vi "HFRR ADV v06.vi"() -> ()   [LabVIEW 2025] (continued)
                        w3346 = dbl[] [] ("History Data")
                        w3347 = cluster{"y":dbl, dbl, "y":dbl}[] [] ("History Data")
                        w3348 = FALSE ("Visible")
                        n2284 = property on="Stroke ( mm )" class="WFChart (strict)"("History Data"=w3347) -> ()  [unwired: 2 in, 2 out]
                        n2285 = property on="Humidity ( %RH )" class="WFChart (strict)"("History Data"=w3346) -> ()  [unwired: 2 in, 2 out]
                        n2286 = property on="Temperature ( Deg C )" class="WFChart (strict)"("History Data"=w3346) -> ()  [unwired: 2 in, 2 out]
                        n2287 = property on="Electrical Contact Resistance ( % )" class="WFChart (strict)"("History Data"=w3346) -> ()  [unwired: 2 in, 2 out]
                        n2288 = property on="Coefficient of Friction" class="WFChart (strict)"("History Data"=w3346) -> ()  [unwired: 2 in, 2 out]
                        n2289 = property on="Frictional Force ( N )" class="WFChart (strict)"("History Data"=w3346) -> ()  [unwired: 2 in, 2 out]
                        n2290 = property on="Coefficient of Friction" class="WFChart (strict)"("History Data"=w3346) -> ()  [unwired: 2 in, 2 out]
                        n2291 = property on="Frictional Force ( N )" class="WFChart (strict)"("History Data"=w3346) -> ()  [unwired: 2 in, 2 out]
                        n2292 = property on="Electrical Contact Resistance ( % )" class="WFChart (strict)"("History Data"=w3346) -> ()  [unwired: 2 in, 2 out]
                        n2293 = property on="Humidity ( %RH )" class="WFChart (strict)"("History Data"=w3346) -> ()  [unwired: 2 in, 2 out]
                        n2294 = property on="Stroke ( mm )" class="WFChart (strict)"("History Data"=w3347) -> ()  [unwired: 2 in, 2 out]
                        n2295 = property on="Temperature ( Deg C )" class="WFChart (strict)"("History Data"=w3346) -> ()  [unwired: 2 in, 2 out]
                        n2296 = property on="Service Password Log" class="Str"("Visible"=w3348) -> ()  [unwired: 2 in, 2 out]
                        n2297 = property on="Password 3" class="Clust (strict)"("Visible"=w3348) -> ()  [unwired: 2 in, 2 out]
                      }
                    }
                    "TEST FILE NAM,E SAVED" <- TRUE ("TEST FILE NAM,E SAVED")
                  }
                }
              }
            }
          }
        }
        n2298 = case shown="True" w2660 {
          frame False {
            n2299 = local write "tfalg"(0.0 ("tfalg")) -> ()
          }
          frame True {
            n2300 = local read "tfalg"() -> (w2805:dbl)
            n2301 = Equal?(x=w2805, y=0.0) -> (x = y?=w2806:bool)
            n2302 = case shown="True" w2806 {
              frame False {
              }
              frame True {
                n2303 = local read "Total No. of Tests"() -> (w2809:dbl)
                n2304 = local write "tfalg"(1.0 ("tfalg")) -> ()
                n2305 = local write "acq 2"(FALSE ("acq 2")) -> ()
                n2306 = Wait (ms)(milliseconds to wait=u32 200) -> ()  [unwired: 1 out]
                n2307 = Increment(x=w2809) -> (x+1=w2808:dbl)
                n2308 = local write "Total No. of Tests"(w2808) -> ()
              }
            }
          }
        }
        n2309 = local write "Test \nStatus"(w2666) -> ()
        n2310 = local write "Save"(w2666) -> ()
        n2311 = local read "Main Tab"() -> (w2623:T2)
        n2312 = case shown="True" w2647 {
          tunnel: [FALSE ("RUN") TRUE ("RUN")] -> w2646
          tunnel: [_ 1] -> w2639
          frame False {
          }
          frame True {
          }
        }
        n2313 = In Range and Coerce(upper limit=w2654, x=w2627, lower limit=w2653) -> (In Range?=w2645:bool)  [unwired: 1 out]
        n2314 = In Range and Coerce(upper limit=w2651, x=w2626, lower limit=w2652) -> (In Range?=w2643:bool)  [unwired: 1 out]
        n2315 = case shown="True" w2659 {
          frame False {
            n2316 = local read "Rt 3"() -> (w2787:bool)
            n2317 = case shown="True" w2787 {
              frame False {
              }
              frame True {
                n2318 = local write "Rt 3"(FALSE ("Rt 3")) -> ()
                n2319 = local write "Json End Flg"(TRUE ("Upld AR 2")) -> ()
              }
            }
            "Rt" <- TRUE ("Rt")
            "Rt 2" <- FALSE ("Rt")
          }
          frame True {
            n2320 = local read "Rt"() -> (w2794:bool)
            n2321 = local write "Rt 2"(TRUE ("Rt 2")) -> ()
            n2322 = case shown="True" w2794 {
              frame False {
              }
              frame True {
                w2795 = TRUE ("Upld AR 2")
                n2323 = local write "Rt"(FALSE ("Rt")) -> ()
                n2324 = local write "Upld AR"(w2795) -> ()
                n2325 = local write "Json St Flg"(w2795) -> ()
              }
            }
            "Rt 3" <- TRUE ("Rt 3")
          }
        }
        n2326 = case shown="True" w2645 {
          tunnel: [FALSE ("RUN") TRUE ("RUN")] -> w2644
          tunnel: [_ 2] -> w2638
          frame False {
          }
          frame True {
          }
        }
        n2327 = case shown="True" w2643 {
          tunnel: [FALSE ("RUN") TRUE ("RUN")] -> w2642
          tunnel: [_ 3] -> w2637
          frame False {
          }
          frame True {
          }
        }
        n2328 = case shown="\"Acquire\"" w2623 {
          tunnel: w2625 -> [_ w2856]
          frame Default {
            w2855 = 0.0 ("output")
            n2329 = local write "PID-out"(w2855) -> ()
            n2330 = local write "Frequency ( Hz )"(w2855) -> ()
          }
          frame "Acquire" {
            n2331 = stacked-sequence {
              frame #0 {
                n2332 = local read "Auto Start Test"() -> (w2861:bool)
                n2333 = case shown="True" w2861 {
                  tunnel: "RUN" -> [w2881 w2884]
                  tunnel: [w2881 w2883] -> w2862
                  frame False {
                  }
                  frame True {
                    n2334 = local read "Auto Start Temp"() -> (w2882:bool)
                    n2335 = Or(x=w2884, y=w2882) -> (x .or. y?=w2883:bool)
                  }
                }
                n2336 = local read "clk"() -> (w2880:dbl)
                n2337 = local read "Save"() -> (w2876:bool)
                n2338 = Equal?(x=w2880, y=0.0) -> (x = y?=w2877:bool)
                n2339 = And(x=w2877, y=w2876) -> (x .and. y?=w2878:bool)
                n2340 = Not(x="Engage") -> (.not. x?=w2867:bool)
                n2341 = case shown="True" w2862 {
                  tunnel: [0.0 w2901] -> w2859
                  frame False {
                    (unwired) TRUE ("Visible")
                    n2342 = local read "Auto Start Test"() -> (w2888:bool)
                    n2343 = local write "Start Time"(TRUE ("Start Time")) -> ()
                    n2344 = property on="Stroke 2" class="DigNum (strict)"("Visible"=FALSE) -> ()  [unwired: 2 in, 2 out]
                    n2345 = case shown="False" w2888 {
                      frame False {
                        n2346 = property on="Heater Button" class="Bool (strict)"("DisabledEnum"=T15."Enabled" ("Disabled")) -> ()  [unwired: 2 in, 2 out]
                        n2347 = property on="Humidity" class="Bool (strict)"("DisabledEnum"=T15."Enabled" ("Disabled")) -> ()  [unwired: 2 in, 2 out]
                      }
                      frame True {
                      }
                    }
                    n2348 = case shown="False" "TestCompFlg" {
                      frame False {
                        n2349 = local read "StartFlg"() -> (w2896:bool)
                        n2350 = case shown="True" w2896 {
                          frame False {
                          }
                          frame True {
                            n2351 = flat-sequence {
                              frame #0 {
                                n2352 = local read "EVENT LOG"() -> (w2898:string)
                                n2353 = call "Event Log.vi"("Content"="Test was interrupted", "EVENT LOG"=w2898) -> ("EVENT LOG"=w2899:string)  [unwired: 8 in, 1 out]
                                n2354 = local write "EVENT LOG"(w2899) -> ()
                              }
                              frame #1 {
                                w2900 = FALSE ("StartFlg")
                                n2355 = local write "Heater Button"(w2900) -> ()
                                n2356 = local write "StartFlg"(w2900) -> ()
                                n2357 = local write "Humidity"(w2900) -> ()
                              }
                            }
                          }
                        }
                      }
                      frame True {
                      }
                    }
                    n2358 = local write "String 14"("Test will autostart once parameters reach the set value." ("String 14")) -> ()
                  }
                  frame True {
                    (unwired) FALSE ("Visible")
                    n2359 = property on="Stroke 2" class="DigNum (strict)"("Visible"=TRUE) -> ()  [unwired: 2 in, 2 out]
                    n2360 = property on="STOP 2" class="Bool (strict)"("Disabled"=u8 2) -> ()  [unwired: 2 in, 2 out]
                    n2361 = local write "String 14"(" Running....." ("String 14")) -> ()
                    n2362 = property on="Heater Button" class="Bool (strict)"("DisabledEnum"=T15."Disabled and Grayed Out" ("Disabled")) -> ()  [unwired: 2 in, 2 out]
                    n2363 = property on="Humidity" class="Bool (strict)"("DisabledEnum"=T15."Disabled and Grayed Out" ("Disabled")) -> ()  [unwired: 2 in, 2 out]
                    n2364 = case shown="True" "Start Time" {
                      selector: "Start Time" -> [_ w2914]
                      frame False {
                      }
                      frame True {
                        n2365 = Not(x=w2914) -> (.not. x?=w2913:bool)
                        n2366 = local write "Start Time"(w2913) -> ()
                        n2367 = local read "EVENT LOG"() -> (w2915:string)
                        n2368 = call "Event Log.vi"("Content"="Test in progress", "EVENT LOG"=w2915) -> ("EVENT LOG"=w2917:string)  [unwired: 8 in, 1 out]
                        n2369 = local write "EVENT LOG"(w2917) -> ()
                      }
                    }
                    n2370 = local read "Set Hz"() -> (w2911:dbl)
                    n2371 = call <vilib>:"Uniform White Noise Waveform.vi"() -> ("signal out"=w2910:waveform(dbl))  [unwired: 10 in, 1 out]
                    n2372 = Add(x=w2911, y=w2910) -> (x+y=w2909:waveform(dbl))
                    n2373 = Multiply(x=w2909, y=ext 0.1) -> (x*y=w2901:waveform(ext))
                    "StartFlg" <- TRUE ("StartFlg")
                  }
                }
                n2374 = case shown="True" w2878 {
                  frame False {
                  }
                  frame True {
                    n2375 = local write "clk"(10.0 ("clk")) -> ()
                    n2376 = Get Date/Time In Seconds() -> (seconds since 1Jan1904=w2920:timestamp)
                    n2377 = To Double Precision Float(number=w2920) -> (double precision float=w2918:dbl)
                    n2378 = local write "acq timer"(w2918) -> ()
                    n2379 = local write "act save time"(w2918) -> ()
                  }
                }
                n2380 = call "Elapsed Time"("Time Target (s)"="Countdown", "Reset"=w2867) -> ("Elapsed Time (s)"=w2872:dbl, "Time has Elapsed"=w2870:bool)  [unwired: 10 in, 6 out]
                "Countdown 2" <- w2872
                n2381 = Subtract(x=w2872, y=2.0) -> (x-y=w2875:dbl)
                n2382 = Less?(x=w2875, y="Countdown") -> (x < y?=w2873:bool)
                n2383 = And(x=w2873, y=w2870) -> (x .and. y?=w2869:bool)
                n2384 = case shown="True" w2869 {
                  frame False {
                  }
                  frame True {
                    (unwired) dbl[] [] ("History Data")
                    n2385 = local write "Engage"(FALSE ("Engage")) -> ()
                    n2386 = local write "RUN"(TRUE ("RUN")) -> ()
                    n2387 = local read "Humidity ( %RH )"() -> (→"Rh Before":dbl)
                  }
                }
                n2388 = local read "Test \nStatus"() -> (w2865:bool)
                n2389 = Multiply(x=w2859, y=10.0) -> (x*y=w2860:dbl)
                n2390 = Select(t=w2860, s=w2865, f=0.0) -> (s? t:f=w2864:dbl)
                n2391 = local write "Frequency ( Hz )"(w2864) -> ()
              }
              frame #1 {
                w2943 = 1000000.0 ("x")
                # "Elapsed time\ncof\nstroke\nAir temp\nTemp\nHumidity"
                # "acq timer\n\nact save time"
                # "convert to microseconds"
                n2392 = local read "COUNT"() -> (w2926:i32)
                n2393 = local read "Rate"() -> (w2939:dbl)
                n2394 = Divide(x=w2943, y=w2939) -> (x/y=w2944:dbl)
                n2395 = Greater Or Equal?(x=w2926, y=250) -> (x >= y?=w2925:bool)
                n2396 = Get Date/Time In Seconds() -> (seconds since 1Jan1904=w2946:timestamp)
                n2397 = case shown="True" w2925 {
                  frame False {
                    n2398 = local read "COUNT"() -> (w2947:i32)
                    n2399 = Increment(x=w2947) -> (x+1=w2948:i32)
                    n2400 = local write "COUNT"(w2948) -> ()
                  }
                  frame True {
                    n2401 = local write "COUNT"(0 ("COUNT")) -> ()
                  }
                }
                n2402 = local read "Samplingtime 2"() -> (w2924:dbl)
                n2403 = local read "act save time"() -> (w2941:dbl)
                n2404 = Divide(x=w2944, y=w2943) -> (x/y=w2942:dbl)
                n2405 = To Double Precision Float(number=w2946) -> (double precision float=w2935:dbl)
                n2406 = Add(x=w2941, y=w2924) -> (x+y=w2940:dbl)
                n2407 = local read "acq timer"() -> (w2945:dbl)
                n2408 = local read "COUNT"() -> (w2928:i32)
                n2409 = Greater Or Equal?(x=w2935, y=w2940) -> (x >= y?=w2923:bool)
                n2410 = Multiply(x=w2942, y=w2928) -> (x*y=w2934:dbl)
                n2411 = Subtract(x=w2935, y=w2945) -> (x-y=w2937:dbl)
                n2412 = local read "Save"() -> (w2938:bool)
                n2413 = Add(x=w2937, y=w2934) -> (x+y=w2921:dbl)
                "Elapsed time 3" <- w2921
                n2414 = And(x=w2923, y=w2938) -> (x .and. y?=w2936:bool)
                n2415 = Divide(x=w2921, y=60.0) -> (x/y=w2932:dbl)
                n2416 = local read "Test \nStatus"() -> (w2922:bool)
                n2417 = local read "clk"() -> (w2929:dbl)
                n2418 = Equal?(x=w2929, y=10.0) -> (x = y?=w2931:bool)
                n2419 = case shown="True" w2936 {
                  tunnel: w2935 -> [_ w3052]
                  tunnel: [FALSE ("Boolean 2") TRUE ("Boolean 2")] -> _
                  frame False {
                  }
                  frame True {
                    w3006 = ";" ("Substring")
                    # "Pid out/\nFreq response value"
                    n2420 = local write "act save time"(w3052) -> ()
                    n2421 = local read "FILE"() -> (w3000:string)
                    n2422 = call "file check.vi"("file name in"=w3000) -> ("error out"=w3003:errorcluster, "file name out"=w2998:string)  [unwired: 9 in]
                    n2423 = call "FILE PATH CREATION.vi"("error in"=w3003, "FILE NAME :"=w2998) -> ("FILE OUT"=w3001:path)  [unwired: 8 in, 1 out]
                    n2424 = Concatenate Strings(w2998, ".dgf" ("Substring")) -> (w3002:string)
                    n2425 = local read "FF 2"() -> (→"Frictional Force ( N )" →"Frictional Force ( N )":dbl)
                    n2426 = Build Path(base path=w3001, name or relative path=w3002) -> (appended path=w2997:path)
                    n2427 = local read "COF 2"() -> (w3011:dbl)
                    "cof" <- w3011
                    "Coefficient of Friction" <- w3011
                    "COF 4" <- w3011
                    "Coefficient of Friction" <- w3011
                    n2428 = local read "TEMP"() -> (w3014:dbl)
                    "Temp" <- w3014
                    "Temperature ( Deg C )" <- w3014
                    n2429 = local read "Humidity ( %RH )"() -> (w3013:dbl)
                    "Humidity ( %RH )" <- w3013
                    "Humidity ( %RH )" <- w3013
                    n2430 = local read "Frequency ( Hz )"() -> (w3020:dbl)
                    n2431 = local read "Elapsed time"() -> (w3045:dbl)
                    n2432 = local read "AIR TEMP"() -> (w3018:dbl)
                    n2433 = local read "PID-out"() -> (w3023:dbl)
                    n2434 = local write "Temperature ( Deg C )"(w3014) -> ()
                    n2435 = Number To Fractional String(number="measured_stroke", width (-)=i16 9 ("precision (6)"), precision (6)=i16 6) -> (F-format string=w3038:string)  [unwired: 1 in]
                    n2436 = Number To Fractional String(number=w3018, width (-)=i16 9 ("precision (6)"), precision (6)=i16 3) -> (F-format string=w3037:string)  [unwired: 1 in]
                    n2437 = Number To Fractional String(number=w3014, width (-)=i16 9 ("precision (6)"), precision (6)=i16 3) -> (F-format string=w3034:string)  [unwired: 1 in]
                    n2438 = Number To Fractional String(number=w3013, width (-)=i16 9 ("precision (6)"), precision (6)=i16 3) -> (F-format string=w3031:string)  [unwired: 1 in]
                    n2439 = Number To Fractional String(number=0.0, width (-)=i16 9 ("precision (6)"), precision (6)=i16 3) -> (F-format string=w3028:string)  [unwired: 1 in]
                    n2440 = Number To Fractional String(number=w3023, width (-)=i16 9 ("precision (6)"), precision (6)=i16 3) -> (F-format string=w3024:string)  [unwired: 1 in]
                    n2441 = Number To Fractional String(number=w3020, width (-)=i16 9 ("precision (6)"), precision (6)=i16 3) -> (F-format string=w3019:string)  [unwired: 1 in]
                    n2442 = Number To Fractional String(number=w3011, width (-)=i16 9 ("precision (6)"), precision (6)=i16 6) -> (F-format string=w3046:string)  [unwired: 1 in]
                    n2443 = Number To Fractional String(number=w3045, width (-)=i16 14 ("precision (6)"), precision (6)=i16 3) -> (F-format string=w3047:string)  [unwired: 1 in]
                    n2444 = Bundle("y"=1.02, "measured_stroke"="measured_stroke", "y"=0.98) -> (w3012:cluster{"y":dbl, "measured_stroke":dbl, "y":dbl})  [unwired: 1 in]
                    n2445 = Number To Fractional String(number="Ambient Humidity :", width (-)=i16 9 ("precision (6)"), precision (6)=i16 6) -> (F-format string=w3004:string)  [unwired: 1 in]
                    n2446 = local read "RUN"() -> (w3010:bool)
                    n2447 = case shown="True" w3010 {
                      tunnel: w3012 -> [_ w3057]
                      tunnel: "measured_stroke" -> [_ w3056]
                      tunnel: "measured_stroke" -> [_ w3055]
                      tunnel: "measured_stroke" -> [_ w3054]
                      frame False {
                      }
                      frame True {
                        "Stroke ( mm )" <- w3057
                        "Stroke ( mm )" <- w3057
                        "Stroke 4" <- w3056
                        "Stroke 3" <- w3055
                        "Stroke 2" <- w3054
                      }
                    }
                    n2448 = Concatenate Strings(w3047, w3006, w3046, w3006, w3038, w3006, w3037, w3006, w3034, w3006, w3031, w3006, w3028, w3006, w3024, w3006, w3019, w3006, w3004, "\r") -> (w3044:string)
                    n2449 = call <vilib>:"Write Characters To File.vi"("append to file? (new file:F)"=TRUE, "character string"=w3044, "file path (dialog if empty)"=w2997) -> ()  [unwired: 2 in, 1 out]
                    "refresh flag" <- TRUE ("refresh flag")
                  }
                }
                n2450 = case shown="True" w2922 {
                  tunnel: w2932 -> [_ w2958]
                  tunnel: w2937 -> [_ w2968]
                  tunnel: [0.0 w2964] -> _
                  tunnel: w2931 -> [_ w2963]
                  tunnel: [0.0 w2962] -> _
                  tunnel: w2921 -> [_ w2962]
                  tunnel: w2935 -> [w2951 _]
                  frame False {
                    n2451 = local write "acq timer"(w2951) -> ()
                    n2452 = local write "Test Duration Status"(0.0 ("Test Duration Status")) -> ()
                  }
                  frame True {
                    n2453 = local read "Set Hz"() -> (w2965:dbl)
                    n2454 = local write "Elapsed time"(w2958) -> ()
                    n2455 = local read "test time"() -> (w2957:dbl)
                    n2456 = Multiply(x=w2968, y=w2965) -> (x*y=w2967:dbl)
                    n2457 = case shown="False" w2963 {
                      tunnel: w2967 -> [w2969 _]
                      tunnel: [w2969 1.0] -> w2964
                      frame False {
                        n2458 = local write "Cycles elapsed"(w2969) -> ()
                      }
                      frame True {
                      }
                    }
                    n2459 = Greater?(x=w2958, y=w2957) -> (0:w2966:bool)
                    n2460 = Subtract(x=w2957, y=w2958) -> (x-y=w2956:dbl)
                    "time" <- w2956
                    n2461 = Multiply(x=w2956, y=60.0) -> (x*y=w2955:dbl)
                    n2462 = local write "Time Remaining"(w2955) -> ()
                    n2463 = local write "Remaining Time"(w2955) -> ()
                    n2464 = case shown="True" w2966 {
                      frame False {
                      }
                      frame True {
                        n2465 = stacked-sequence {
                          frame #0 {
                            w2974 = T15."Enabled" ("Disabled")
                            w2973 = FALSE ("TEST FILE NAM,E SAVED")
                            w2975 = "" ("FILE")
                            w2976 = TRUE ("Visible")
                            n2466 = local write "Humidity"(FALSE ("Humidity")) -> ()
                            n2467 = local write "RUN"(FALSE ("OK Button 2")) -> ()
                            n2468 = local write "Heater Button"(FALSE ("Heater Button")) -> ()
                            n2469 = local write "Auto Start Test"(FALSE ("Auto Start Test")) -> ()
                            n2470 = local write "TestCompFlg"(TRUE ("StpFlg")) -> ()
                            n2471 = local read "Humidity ( %RH )"() -> (→"Rh After":dbl)
                            n2472 = property on="STOP 2" class="Bool (strict)"("Disabled"=u8 0) -> ()  [unwired: 2 in, 2 out]
                            n2473 = local read "EVENT LOG"() -> (w2981:string)
                            n2474 = call "Event Log.vi"("Content"="Test Completed", "EVENT LOG"=w2981) -> ("EVENT LOG"=w2980:string)  [unwired: 8 in, 1 out]
                            n2475 = property on="RUN" class="Bool (strict)"("Visible"=w2976) -> ()  [unwired: 2 in, 2 out]
                            n2476 = property on="Auto Start Test" class="Bool (strict)"("Visible"=w2976) -> ()  [unwired: 2 in, 2 out]
                            n2477 = local write "Batch Ref Num :"(w2975) -> ()
                            n2478 = local write "FILE"(w2975) -> ()
                            n2479 = local write "EVENT LOG"(w2980) -> ()
                            n2480 = local write "TEST FILE NAM,E SAVED"(w2973) -> ()
                            n2481 = local write "Fuel Discription :"(w2975) -> ()
                            n2482 = local write "START TEMP"(w2973) -> ()
                            n2483 = local write "Remarks :"(w2975) -> ()
                            n2484 = local write "Main Dashboard Buttons"(T1."Imaging" ("Main Dashboard Buttons")) -> ()
                            n2485 = local write "Main Tab"(T2."Adv Scar" ("Main Tab")) -> ()
                            n2486 = property on="FRICVALZ 2" class="Bool (strict)"("DisabledEnum"=w2974) -> ()  [unwired: 2 in, 2 out]
                            n2487 = property on="FRICVALZ 3" class="Bool (strict)"("DisabledEnum"=w2974) -> ()  [unwired: 2 in, 2 out]
                            n2488 = property on="FRICVALZ 4" class="Bool (strict)"("DisabledEnum"=w2974) -> ()  [unwired: 2 in, 2 out]
                          }
                          frame #1 {
                            n2489 = Wait (ms)(milliseconds to wait=u32 1500) -> ()  [unwired: 1 out]
                          }
                          frame #2 {
                            n2490 = local write "Command"("VC;0") -> ()
                          }
                          frame #3 {
                            n2491 = Wait (ms)(milliseconds to wait=u32 1500) -> ()  [unwired: 1 out]
                          }
                          frame #4 {
                            n2492 = local write "Command"("ST;0") -> ()
                          }
                          frame #5 {
                            n2493 = Wait (ms)(milliseconds to wait=u32 1500) -> ()  [unwired: 1 out]
                          }
                          frame #6 {
                            n2494 = local write "Command"("HE;0" ("Command")) -> ()
                          }
                          frame #7 {
                            n2495 = Wait (ms)(milliseconds to wait=u32 1500) -> ()  [unwired: 1 out]
                          }
                        }
                      }
                    }
                    n2496 = Divide(x=w2958, y=w2957) -> (x/y=w2961:dbl)
                    n2497 = Multiply(x=w2961, y=100.0) -> (x*y=w2959:dbl)
                    n2498 = local write "Test Duration Status"(w2959) -> ()
                  }
                }
              }
              frame #2 {
                n2499 = case shown="True" "Heater Button" {
                  tunnel: [0.0 ("output") w3067] -> w3058
                  frame False {
                    w3061 = TRUE ("tmpchk")
                    n2500 = local read "TEMP"() -> (w3062:dbl)
                    n2501 = local write "Temp ini"(w3062) -> ()
                    n2502 = local write "Reset 4"(w3061) -> ()
                    n2503 = local write "tmpchk"(w3061) -> ()
                    n2504 = local write "reinit"(TRUE ("reinit")) -> ()
                    n2505 = local write "manual temp log"(TRUE ("manual temp log")) -> ()
                  }
                  frame True {
                    n2506 = local read "Auto Start Test"() -> (w3066:bool)
                    n2507 = case shown="True" FALSE {
                      tunnel: [_ w3082] -> w3067
                      frame False {
                      }
                      frame True {
                        # "Logic to turn off\nthe heater when \ntemp is not rising.\nTime - 60 sec\nDelta t- 5°c"
                        n2508 = local read "Temp ini"() -> (w3071:dbl)
                        n2509 = Less?(x=w3071, y=53.0) -> (x < y?=w3069:bool)
                        n2510 = And(x="tmpchk", y=w3069) -> (x .and. y?=w3072:bool)
                        n2511 = case shown="True" w3072 {
                          frame False {
                          }
                          frame True {
                            n2512 = call "Elapsed Time8"("Time Target (s)"=300.0, "Reset"="Reset 4") -> ("Time has Elapsed"=w3085:bool)  [unwired: 10 in, 7 out]
                            n2513 = flat-sequence {
                              tunnel: w3085 -> [_]
                              frame #0 {
                                n2514 = local write "Reset 4"(FALSE ("Reset 4")) -> ()
                              }
                            }
                            n2515 = case shown="True" w3085 {
                              frame False {
                              }
                              frame True {
                                n2516 = local read "Temp ini"() -> (w3092:dbl)
                                n2517 = Add(x=w3092, y=5.0) -> (x+y=w3090:dbl)
                                n2518 = local read "TEMP"() -> (w3093:dbl)
                                n2519 = Greater?(x=w3093, y=w3090) -> (0:w3091:bool)
                                n2520 = case shown="False" w3091 {
                                frame False {
                                n2521 = local write "Heater Button"(FALSE ("Heater Button")) -> ()
                                }
                                frame True {
                                n2522 = local write "tmpchk"(FALSE ("tmpchk")) -> ()
                                }
                                }
                              }
                            }
                          }
                        }
                        n2523 = local read "Set Temp"() -> (w3080:dbl)
                        n2524 = local read "TEMP"() -> (w3074:dbl)
                        n2525 = call-poly <vilib>:"PID.vi"("reinitialize? (F)"="reinit", "dt (s)"=-1.0, "process variable"=w3074, "setpoint"=w3080) -> ("output"=w3077:dbl)  [unwired: 6 in, 1 out]
                        n2526 = Subtract(x=w3080, y=w3074) -> (x-y=w3081:dbl)
                        n2527 = Add(x=w3080, y=0.5) -> (x+y=w3078:dbl)
                        n2528 = Greater Or Equal?(x=w3074, y=w3078) -> ()  [unwired: 1 out]
                        n2529 = Select(t=0.0, s=FALSE, f=w3077) -> (s? t:f=w3076:dbl)
                        "PID output" <- w3076
                        n2530 = flat-sequence {
                          tunnel: w3076 -> [w3096]
                          tunnel: [w3096] -> w3082
                          frame #0 {
                            n2531 = local write "reinit"(FALSE ("reinit")) -> ()
                          }
                        }
                        n2532 = Bundle(w3081, "output"=w3076, "TEMP"=w3074) -> ()  [unwired: 1 in, 1 out]
                      }
                    }
                    n2533 = case shown="False" w3066 {
                      frame False {
                        n2534 = local read "Set Temp"() -> (w3104:dbl)
                        n2535 = local read "TEMP"() -> (w3103:dbl)
                        n2536 = Subtract(x=w3104, y=w3103) -> (x-y=w3102:dbl)
                        n2537 = Absolute Value(x=w3102) -> (abs(x)=w3101:dbl)
                        n2538 = Less?(x=w3101, y=0.5) -> (x < y?=w3099:bool)
                        n2539 = case shown="True" w3099 {
                          tunnel: "manual temp log" -> [_ w3105]
                          frame False {
                          }
                          frame True {
                            n2540 = case shown="True" w3105 {
                              selector: w3105 -> [_ w3106]
                              frame False {
                              }
                              frame True {
                                # "#Event log"
                                n2541 = Not(x=w3106) -> (.not. x?=w3107:bool)
                                n2542 = local write "manual temp log"(w3107) -> ()
                                n2543 = local read "EVENT LOG"() -> (w3110:string)
                                n2544 = call "Event Log.vi"("Content"="Target Temperature reached", "EVENT LOG"=w3110) -> ("EVENT LOG"=w3109:string)  [unwired: 8 in, 1 out]
                                n2545 = local write "EVENT LOG"(w3109) -> ()
                              }
                            }
                          }
                        }
                      }
                      frame True {
                        n2546 = local write "manual temp log"(TRUE ("manual temp log")) -> ()
                      }
                    }
                  }
                }
                "PID-out" <- w3058
              }
              frame #3 {
                n2547 = local read "TEMP"() -> (w3112:dbl)
                n2548 = Greater Or Equal?(x=w3112, y="Set Temp 2") -> (x >= y?=w3117:bool)
                n2549 = case shown="True" w3117 {
                  tunnel: [FALSE TRUE] -> w3115
                  frame False {
                  }
                  frame True {
                  }
                }
                "Status 13" <- w3115
                n2550 = And(x=w3115, y="trip1 8") -> (x .and. y?=w3114:bool)
                n2551 = case shown="True" w3114 {
                  frame False {
                    n2552 = local write "Heater Trip Temp"(TRUE ("Heater Trip Temp")) -> ()
                  }
                  frame True {
                    w3120 = FALSE ("OK Button 2")
                    n2553 = case shown="True" "Heater Trip Temp" {
                      selector: "Heater Trip Temp" -> [_ w3122]
                      frame False {
                      }
                      frame True {
                        n2554 = Not(x=w3122) -> (.not. x?=w3121:bool)
                        n2555 = local read "EVENT LOG"() -> (w3125:string)
                        n2556 = local write "Heater Trip Temp"(w3121) -> ()
                        n2557 = call "Event Log.vi"("Content"="Heater Trip", "EVENT LOG"=w3125) -> ("EVENT LOG"=w3124:string)  [unwired: 8 in, 1 out]
                        n2558 = local write "EVENT LOG"(w3124) -> ()
                      }
                    }
                    n2559 = local write "RUN"(w3120) -> ()
                    n2560 = property on="Auto Start Test" class="Bool (strict)"("Value"=w3120) -> ()  [unwired: 2 in, 2 out]
                    n2561 = local write "Heater Button"(w3120) -> ()
                  }
                }
              }
            }
            n2562 = case shown="False" w2856 {
              frame False {
                n2563 = disable-structure shown="Enabled" {
                  frame Disabled {
                    n2564 = stacked-sequence {
                      frame #0 {
                        n2565 = local write "RUN"(FALSE ("OK Button 2")) -> ()
                      }
                      frame #1 {
                      }
                    }
                  }
                  frame Enabled {
                  }
                }
              }
              frame True {
              }
            }
          }
        }
        n2566 = local read "airtempflg"() -> (w2648:bool)
        n2567 = Or(x=w2648, y=w2646) -> (x .or. y?=w2649:bool)
        n2568 = Insert Into Array(array=string[] ["Air Temperature has reached set value,", "Humidity has reached set value,", "Sample Temperaturehas reached set value,", ""], index=0, new element="") -> (w2634:string[])
        n2569 = Build Array(w2639, w2638, w2637) -> (w2635:i32[])
        n2570 = disable-structure shown="Disabled" {
          disable-tunnel: w2649 -> [w2726 _]
          disable-tunnel: w2644 -> [w2725 _]
          disable-tunnel: w2642 -> [w2724 _]
          frame Disabled {
            n2571 = Compound Arithmetic op=AND(w2726, w2725, w2724) -> ()  [unwired: 1 out]
            n2572 = case shown="True" {
              selector: _ -> [_ _]
              frame False {
              }
              frame True {
                w2727 = FALSE ("autostrtflg")
                n2573 = local write "RUN"(TRUE ("RUN")) -> ()
                n2574 = local write "autostrtflg"(w2727) -> ()
                n2575 = local write "autostart"(w2727) -> ()
                n2576 = local write "String 14"(" Running....." ("String 14")) -> ()
              }
            }
          }
          frame Enabled {
          }
        }
        n2577 = for {
          tunnel: w2635 -> [w2777] mode=indexing
          tunnel: w2634 -> [w2776]
          shift-right: [w2773] -> w2633
          shift-left: "" -> [w2775]
          n2578 = Index Array(array=w2776, index=w2777) -> (element=w2774:string)
          n2579 = Concatenate Strings(w2774, w2775) -> (w2773:string)
        }
        n2580 = local write "autostart 2"(w2633) -> ()
        n2581 = local read "Reset Graph"() -> (w2622:bool)
        n2582 = case shown="True" w2622 {
          selector: w2622 -> [_ w2676]
          frame False {
          }
          frame True {
            w2690 = 0.0 ("X Scale.Range:Maximum")
            n2583 = Not(x=w2676) -> (.not. x?=w2675:bool)
            n2584 = local write "Reset Graph"(w2675) -> ()
            n2585 = property on="Electrical Contact Resistance ( % )" class="WFChart (strict)"("XScale.Maximum"=600.0 ("X Scale.Range:Maximum"), "XScale.Minimum"=0.0 ("X Scale.Range:Minimum"), "YScale.Maximum"=100.0 ("Y Scale.Range:Maximum"), "YScale.Minimum"=0.0 ("Y Scale.Range:Minimum")) -> ()  [unwired: 2 in, 2 out]
            n2586 = property on="Frictional Force ( N )" class="WFChart (strict)"("XScale.Maximum"=600.0 ("X Scale.Range:Maximum"), "XScale.Minimum"=0.0 ("X Scale.Range:Minimum"), "YScale.Maximum"=100.0 ("Y Scale.Range:Maximum"), "YScale.Minimum"=0.0 ("Y Scale.Range:Minimum")) -> ()  [unwired: 2 in, 2 out]
            n2587 = property on="Temperature ( Deg C )" class="WFChart (strict)"("XScale.Maximum"=600.0 ("X Scale.Range:Maximum"), "XScale.Minimum"=0.0 ("X Scale.Range:Minimum"), "YScale.Maximum"=100.0 ("Y Scale.Range:Maximum"), "YScale.Minimum"=0.0 ("Y Scale.Range:Minimum")) -> ()  [unwired: 2 in, 2 out]
            n2588 = property on="Humidity ( %RH )" class="WFChart (strict)"("XScale.Maximum"=600.0 ("X Scale.Range:Maximum"), "XScale.Minimum"=0.0 ("X Scale.Range:Minimum"), "YScale.Maximum"=100.0 ("Y Scale.Range:Maximum"), "YScale.Minimum"=0.0 ("Y Scale.Range:Minimum")) -> ()  [unwired: 2 in, 2 out]
            n2589 = property on="Stroke ( mm )" class="WFChart (strict)"("XScale.Maximum"=600.0 ("X Scale.Range:Maximum"), "XScale.Minimum"=0.0 ("X Scale.Range:Minimum"), "YScale.Maximum"=100.0 ("Y Scale.Range:Maximum"), "YScale.Minimum"=0.0 ("Y Scale.Range:Minimum")) -> ()  [unwired: 2 in, 2 out]
            n2590 = property on="Coefficient of Friction" class="WFChart (strict)"("XScale.Maximum"=600.0 ("X Scale.Range:Maximum"), "XScale.Minimum"=0.0 ("X Scale.Range:Minimum"), "YScale.Maximum"=100.0 ("Y Scale.Range:Maximum"), "YScale.Minimum"=0.0 ("Y Scale.Range:Minimum")) -> ()  [unwired: 2 in, 2 out]
            n2591 = property on="Electrical Contact Resistance ( % )" class="WFChart (strict)"("XScale.Minimum"=0.0 ("X Scale.Range:Minimum"), "XScale.Maximum"=600.0 ("X Scale.Range:Maximum"), "YScale.Minimum"=0.0 ("Y Scale.Range:Minimum"), "YScale.Maximum"=100.0 ("Y Scale.Range:Maximum")) -> ()  [unwired: 2 in, 2 out]
            n2592 = property on="Temperature ( Deg C )" class="WFChart (strict)"("XScale.Minimum"=0.0 ("X Scale.Range:Minimum"), "XScale.Maximum"=600.0 ("X Scale.Range:Maximum"), "YScale.Minimum"=0.0 ("Y Scale.Range:Minimum"), "YScale.Maximum"=100.0 ("Y Scale.Range:Maximum")) -> ()  [unwired: 2 in, 2 out]
            n2593 = property on="Coefficient of Friction" class="WFChart (strict)"("XScale.Minimum"=0.0 ("X Scale.Range:Minimum"), "XScale.Maximum"=600.0 ("X Scale.Range:Maximum"), "YScale.Maximum"=1.0 ("X Scale.Range:Minimum"), "YScale.Minimum"=0.0 ("X Scale.Range:Minimum")) -> ()  [unwired: 2 in, 2 out]
            n2594 = property on="Frictional Force ( N )" class="WFChart (strict)"("XScale.Maximum"=600.0 ("X Scale.Range:Maximum"), "XScale.Minimum"=w2690, "YScale.Maximum"=10.0 ("Y Scale.Range:Maximum"), "YScale.Minimum"=w2690) -> ()  [unwired: 2 in, 2 out]
            n2595 = property on="Stroke ( mm )" class="WFChart (strict)"("XScale.Maximum"=600.0 ("X Scale.Range:Maximum"), "XScale.Minimum"=0.0 ("X Scale.Range:Minimum"), "YScale.Maximum"=100.0 ("Y Scale.Range:Maximum"), "YScale.Minimum"=0.0 ("Y Scale.Range:Minimum")) -> ()  [unwired: 2 in, 2 out]
            n2596 = property on="Humidity ( %RH )" class="WFChart (strict)"("XScale.Maximum"=600.0 ("X Scale.Range:Maximum"), "XScale.Minimum"=0.0 ("X Scale.Range:Minimum"), "YScale.Maximum"=100.0 ("Y Scale.Range:Maximum"), "YScale.Minimum"=0.0 ("Y Scale.Range:Minimum")) -> ()  [unwired: 2 in, 2 out]
          }
        }
      }
      frame "Compare Files" {
        # "Elapsed time\ncof\nstroke\nAir temp\nTemp\nHumidity"
        n2597 = case shown="True" "RSTV1 2" {
          frame False {
          }
          frame True {
            n2598 = property on="Humidity ( %RH )" class="XYGraph (strict)"("Y Scale.Display Format:Precision"=u8 0 ("Y Scale.Format & Precision:Precision")) -> ()  [unwired: 2 in, 2 out]
            n2599 = property on="Humidity ( %RH )" class="XYGraph (strict)"("X Scale.Range:Minimum"=0.0, "X Scale.Range:Maximum"=75.0, "Y Scale.Range:Minimum"=48.0, "Y Scale.Range:Maximum"=58.0) -> ()  [unwired: 2 in, 2 out]
          }
        }
        n2600 = case shown="True" "RST CP 2" {
          frame False {
          }
          frame True {
            n2601 = property on="XY Graph 13" class="XYGraph (strict)"("Y Scale.Display Format:Precision"=u8 0 ("Y Scale.Format & Precision:Precision")) -> ()  [unwired: 2 in, 2 out]
            n2602 = property on="XY Graph 13" class="XYGraph (strict)"("X Scale.Range:Minimum"=0.0, "X Scale.Range:Maximum"=75.0, "Y Scale.Range:Minimum"=0.0, "Y Scale.Range:Maximum"=100.0) -> ()  [unwired: 2 in, 2 out]
          }
        }
        n2603 = case shown="True" "RST CP" {
          frame False {
          }
          frame True {
            n2604 = property on="Sample Temperature ( °C )" class="XYGraph (strict)"("Y Scale.Display Format:Precision"=u8 2 ("Y Scale.Format & Precision:Precision")) -> ()  [unwired: 2 in, 2 out]
            n2605 = property on="Sample Temperature ( °C )" class="XYGraph (strict)"("X Scale.Range:Minimum"=0.0, "X Scale.Range:Maximum"=75.0, "Y Scale.Range:Minimum"=58.0, "Y Scale.Range:Maximum"=62.0) -> ()  [unwired: 2 in, 2 out]
          }
        }
        n2606 = case shown="True" "RSTV1 3" {
          frame False {
          }
          frame True {
            n2607 = property on="Air Temperature  ( °C )" class="XYGraph (strict)"("Y Scale.Display Format:Precision"=u8 2 ("Y Scale.Format & Precision:Precision")) -> ()  [unwired: 2 in, 2 out]
            n2608 = property on="Air Temperature  ( °C )" class="XYGraph (strict)"("X Scale.Range:Minimum"=0.0 ("Y Scale.Range:Minimum"), "X Scale.Range:Maximum"=75.0 ("Y Scale.Range:Maximum"), "Y Scale.Range:Minimum"=20.0 ("X Scale.Range:Minimum"), "Y Scale.Range:Maximum"=26.0 ("X Scale.Range:Maximum")) -> ()  [unwired: 2 in, 2 out]
          }
        }
        n2609 = case shown="True" "RSTV1 4" {
          frame False {
          }
          frame True {
            n2610 = property on="Stroke ( mm )" class="XYGraph (strict)"("Y Scale.Display Format:Precision"=u8 2 ("Y Scale.Format & Precision:Precision")) -> ()  [unwired: 2 in, 2 out]
            n2611 = property on="Stroke ( mm )" class="XYGraph (strict)"("X Scale.Range:Minimum"=0.0 ("Y Scale.Range:Maximum"), "X Scale.Range:Maximum"=75.0 ("X Scale.Range:Minimum"), "Y Scale.Range:Minimum"=0.98, "Y Scale.Range:Maximum"=1.02) -> ()  [unwired: 2 in, 2 out]
          }
        }
        n2612 = case shown="True" "rstv2" {
          frame False {
          }
          frame True {
            n2613 = property on="Coefficient Of Friction" class="XYGraph (strict)"("Y Scale.Display Format:Precision"=u8 3 ("Y Scale.Format & Precision:Precision")) -> ()  [unwired: 2 in, 2 out]
            n2614 = property on="Coefficient Of Friction" class="XYGraph (strict)"("X Scale.Range:Minimum"=0.0 ("Y Scale.Range:Maximum"), "X Scale.Range:Maximum"=75.0, "Y Scale.Range:Minimum"=0.0, "Y Scale.Range:Maximum"=1.0 ("X Scale.Range:Minimum")) -> ()  [unwired: 2 in, 2 out]
          }
        }
        n2615 = case shown="True" "RST CP 3" {
          frame False {
          }
          frame True {
            n2616 = property on="Air Temp ( °C ) vs Humidity ( % RH )" class="XYGraph (strict)"("X Scale.Range:Minimum"=18.0, "X Scale.Range:Maximum"=28.0 ("X Scale.Range:Minimum"), "Y Scale.Range:Minimum"=30.0 ("X Scale.Range:Minimum"), "Y Scale.Range:Maximum"=70.0 ("X Scale.Range:Minimum")) -> ()  [unwired: 2 in, 2 out]
          }
        }
        n2617 = case shown="True" "OPEN 1" {
          frame False {
          }
          frame True {
            (unwired) 0  # existing file
            w3401 = "Choose a datalog file to open"  # prompt
            n2618 = local write "OPEN 1"(FALSE ("OPEN 1")) -> ()
            n2619 = String To Path(string="C:\\LAB-IQ\\Data\\") -> (path=w3386:path)
            n2620 = File Dialog(6:"*.dgf" ("pattern"), 7:w3401, 11:w3386) -> (0:w3384:errorcluster, 3:w3392:path)  [unwired: 4 in, 2 out]
            n2621 = Unbundle(w3384) -> ()  [unwired: 3 out]
            n2622 = Strip Path(path=w3392) -> (name=w3391:string)  [unwired: 1 out]
            n2623 = Path To String(path=w3392) -> (string=w3387:string)
            "string1" <- w3387
            n2624 = Match Pattern(string=w3391, regular expression=".dgf") -> (before substring=→"String Control":string)  [unwired: 1 in, 3 out]
            n2625 = Match Pattern(string=w3387, regular expression=".dgf" ("substring (\"\")")) -> (before substring=w3397:string)  [unwired: 1 in, 3 out]
            n2626 = Concatenate Strings(w3397, ".duf" ("Substring")) -> (w3393:string)
            n2627 = String To Path(string=w3393) -> (path=w3398:path)
            n2628 = call <vilib>:"Read Characters From File.vi"("file path (dialog if empty)"=w3398, "start of read offset (chars.:0)"=60 ("start of read offset (chars.: 0)")) -> ("character string"=→"String Control 2":string)  [unwired: 4 in, 3 out]
          }
        }
        n2629 = case shown="True" "OPEN 2" {
          frame False {
          }
          frame True {
            (unwired) 0  # existing file
            w3419 = "Choose a datalog file to open"  # prompt
            n2630 = local write "OPEN 2"(FALSE ("OPEN 1")) -> ()
            n2631 = String To Path(string="C:\\LAB-IQ\\Data\\") -> (path=w3404:path)
            n2632 = File Dialog(6:"*.dgf" ("pattern"), 7:w3419, 11:w3404) -> (0:w3402:errorcluster, 3:w3410:path)  [unwired: 4 in, 2 out]
            n2633 = Unbundle(w3402) -> ()  [unwired: 3 out]
            n2634 = Strip Path(path=w3410) -> (name=w3408:string)  [unwired: 1 out]
            n2635 = Path To String(path=w3410) -> (string=w3405:string)
            "string1 2" <- w3405
            n2636 = Match Pattern(string=w3408, regular expression=".dgf") -> (before substring=→"String Control 3":string)  [unwired: 1 in, 3 out]
            n2637 = Match Pattern(string=w3405, regular expression=".dgf" ("substring (\"\")")) -> (before substring=w3416:string)  [unwired: 1 in, 3 out]
            n2638 = Concatenate Strings(w3416, ".duf" ("Substring")) -> (w3413:string)
            n2639 = String To Path(string=w3413) -> (path=w3411:path)
            n2640 = call <vilib>:"Read Characters From File.vi"("file path (dialog if empty)"=w3411, "start of read offset (chars.:0)"=60 ("start of read offset (chars.: 0)")) -> ("character string"=→"String Control 4":string)  [unwired: 4 in, 3 out]
          }
        }
        n2641 = case shown="True" "OPEN 3" {
          frame False {
          }
          frame True {
            (unwired) 0  # existing file
            w3437 = "Choose a datalog file to open"  # prompt
            n2642 = local write "OPEN 3"(FALSE ("OPEN 1")) -> ()
            n2643 = String To Path(string="C:\\LAB-IQ\\Data\\") -> (path=w3422:path)
            n2644 = File Dialog(6:"*.dgf" ("pattern"), 7:w3437, 11:w3422) -> (0:w3420:errorcluster, 3:w3428:path)  [unwired: 4 in, 2 out]
            n2645 = Unbundle(w3420) -> ()  [unwired: 3 out]
            n2646 = Strip Path(path=w3428) -> (name=w3426:string)  [unwired: 1 out]
            n2647 = Path To String(path=w3428) -> (string=w3423:string)
            "string1 3" <- w3423
            n2648 = Match Pattern(string=w3426, regular expression=".dgf") -> (before substring=→"String Control 5":string)  [unwired: 1 in, 3 out]
            n2649 = Match Pattern(string=w3423, regular expression=".dgf" ("substring (\"\")")) -> (before substring=w3433:string)  [unwired: 1 in, 3 out]
            n2650 = Concatenate Strings(w3433, ".duf" ("Substring")) -> (w3430:string)
            n2651 = String To Path(string=w3430) -> (path=w3434:path)
            n2652 = call <vilib>:"Read Characters From File.vi"("file path (dialog if empty)"=w3434, "start of read offset (chars.:0)"=60 ("start of read offset (chars.: 0)")) -> ("character string"=→"String Control 6":string)  [unwired: 4 in, 3 out]
          }
        }
        n2653 = case shown="True" "OPEN 4" {
          frame False {
          }
          frame True {
            (unwired) 0  # existing file
            w3455 = "Choose a datalog file to open"  # prompt
            n2654 = local write "OPEN 4"(FALSE ("OPEN 1")) -> ()
            n2655 = String To Path(string="C:\\LAB-IQ\\Data\\") -> (path=w3440:path)
            n2656 = File Dialog(6:"*.dgf" ("pattern"), 7:w3455, 11:w3440) -> (0:w3438:errorcluster, 3:w3446:path)  [unwired: 4 in, 2 out]
            n2657 = Unbundle(w3438) -> ()  [unwired: 3 out]
            n2658 = Strip Path(path=w3446) -> (name=w3444:string)  [unwired: 1 out]
            n2659 = Path To String(path=w3446) -> (string=w3441:string)
            "string1 4" <- w3441
            n2660 = Match Pattern(string=w3444, regular expression=".dgf") -> (before substring=→"String Control 7":string)  [unwired: 1 in, 3 out]
            n2661 = Match Pattern(string=w3441, regular expression=".dgf" ("substring (\"\")")) -> (before substring=w3451:string)  [unwired: 1 in, 3 out]
            n2662 = Concatenate Strings(w3451, ".duf" ("Substring")) -> (w3448:string)
            n2663 = String To Path(string=w3448) -> (path=w3452:path)
            n2664 = call <vilib>:"Read Characters From File.vi"("file path (dialog if empty)"=w3452, "start of read offset (chars.:0)"=60 ("start of read offset (chars.: 0)")) -> ("character string"=→"String Control 8":string)  [unwired: 4 in, 3 out]
          }
        }
      }
      frame "About" {
        # "Elapsed time\ncof\nstroke\nmean pos\nTemp\nHumidity"
        n2665 = disable-structure shown="Disabled" {
          frame Disabled {
            n2666 = case shown="True" "Export" {
              frame False {
              }
              frame True {
                w3477 = "                                      " ("string")
                w3479 = "\r"
                (unwired) i16 6 ("width (-)")
                w3556 = "\r"
                w3488 = "\r"
                n2667 = local write "Export"(FALSE ("Export")) -> ()
                n2668 = local read "String 29"() -> (w3525:string)
                n2669 = local read "String 34"() -> (w3513:string)
                n2670 = local read "String 35"() -> (w3508:string)
                n2671 = local read "String 37"() -> (w3504:string)
                n2672 = local read "String 36"() -> (w3501:string)
                n2673 = local read "String 38"() -> (w3498:string)
                n2674 = local read "String 39"() -> (w3495:string)
                n2675 = Match Pattern(string=w3525, regular expression=".dwm") -> (before substring=w3521:string)  [unwired: 1 in, 3 out]
                "before substring" <- w3521
                n2676 = local read "S 38"() -> (w3516:string)
                n2677 = local read "S 39"() -> (w3509:string)
                n2678 = local read "Temperature before test 2"() -> (w3545:dbl)
                n2679 = local read "Temperature after test 2"() -> (w3550:dbl)
                n2680 = local read "Humidity before test 2"() -> (w3531:dbl)
                n2681 = local read "Humidity after test 2"() -> (w3546:dbl)
                n2682 = local read "MWSD 2"() -> (w3542:dbl)
                n2683 = local read "WS1.4 2"() -> (w3558:dbl)
                n2684 = local read "HCF 2"() -> (w3554:dbl)
                n2685 = local read "AVP 2"() -> (w3543:dbl)
                n2686 = Concatenate Strings("1," ("string"), w3516) -> (w3515:string)
                n2687 = Concatenate Strings("2," ("string"), w3513) -> (w3512:string)
                n2688 = Concatenate Strings("3," ("string"), w3509) -> (w3511:string)
                n2689 = Concatenate Strings("4," ("string"), w3508) -> (w3507:string)
                n2690 = Concatenate Strings("5," ("string"), w3504) -> (w3505:string)
                n2691 = Concatenate Strings("6," ("string"), w3501) -> (w3502:string)
                n2692 = Concatenate Strings("7," ("string"), w3498) -> (w3499:string)
                n2693 = Concatenate Strings("8," ("string"), w3495) -> (w3496:string)
                n2694 = local read "Sample ID"() -> (w3563:string)
                n2695 = case shown="\"xlx\"" "Select File Type" {
                  tunnel: w3521 -> [w3566 w3568 w3570]
                  tunnel: [w3564 w3569 w3571] -> w3520
                  frame "xlx" {
                    n2696 = Concatenate Strings(w3566, ".xls" ("string")) -> (w3564:string)
                  }
                  frame "csv" {
                    n2697 = Concatenate Strings(w3568, ".csv" ("string")) -> (w3569:string)
                  }
                  frame "txt" {
                    n2698 = Concatenate Strings(w3570, ".txt" ("string")) -> (w3571:string)
                  }
                }
                n2699 = local read "Test Date"() -> (w3562:string)
                n2700 = local read "String 45"() -> (w3476:string)
                n2701 = local read "String 31"() -> (w3561:string)
                n2702 = local read "String 32"() -> (w3560:string)
                n2703 = local read "TITTLE"() -> (w3484:string)
                n2704 = Number To Fractional String(number=w3531, width (-)=i16 6, precision (6)=i16 2) -> (F-format string=w3530:string)  [unwired: 1 in]
                n2705 = Number To Fractional String(number=w3545, width (-)=i16 6, precision (6)=i16 2) -> (F-format string=w3551:string)  [unwired: 1 in]
                n2706 = Number To Fractional String(number=w3546, width (-)=i16 6, precision (6)=i16 2) -> (F-format string=w3544:string)  [unwired: 1 in]
                n2707 = Number To Fractional String(number=w3550, width (-)=i16 6, precision (6)=i16 2) -> (F-format string=w3549:string)  [unwired: 1 in]
                n2708 = Number To Fractional String(number=w3542, width (-)=i16 6, precision (6)=i16 2) -> (F-format string=w3540:string)  [unwired: 1 in]
                n2709 = Number To Fractional String(number=w3543, width (-)=i16 6, precision (6)=i16 2) -> (F-format string=w3541:string)  [unwired: 1 in]
                n2710 = Number To Fractional String(number=w3554, width (-)=i16 6, precision (6)=i16 2) -> (F-format string=w3555:string)  [unwired: 1 in]
                n2711 = Number To Fractional String(number=w3558, precision (6)=i16 2) -> (F-format string=w3559:string)  [unwired: 2 in]
                n2712 = local read "s.NO"() -> (w3478:string)
                n2713 = Concatenate Strings("=" ("string"), w3484) -> (w3483:string)
                n2714 = Concatenate Strings("S.No," ("string"), "                                       Parameters" ("string")) -> (w3489:string)
                n2715 = Concatenate Strings(w3556, w3515, w3530, w3556, w3512, w3551, w3556, w3511, w3544, w3556, w3507, w3549, w3556, w3505, w3540, w3556, w3502, w3541, w3556, w3499, w3555, w3556, w3496, w3559) -> (w3518:string)
                n2716 = Concatenate Strings(w3488, "," ("string"), w3476, w3478, w3477, w3560, w3563, w3477, w3561, w3562, w3488) -> (w3486:string)
                n2717 = local read "Tested by"() -> (w3492:string)
                n2718 = local read "String 33"() -> (w3493:string)
                n2719 = Concatenate Strings("," ("string"), "                                                                             " ("string")) -> (w3481:string)
                n2720 = Concatenate Strings(w3483, w3479, w3486, w3479, w3489, w3518, w3479, w3481, w3493, w3492) -> (→"export":string)
                n2721 = String To Path(string=w3520) -> (path=w3527:path)
                n2722 = local read "export"() -> (w3522:string)
                n2723 = call <vilib>:"Write Characters To File.vi"("append to file? (new file:F)"=FALSE, "character string"=w3522, "file path (dialog if empty)"=w3527) -> ()  [unwired: 2 in, 1 out]
              }
